vi "N6705b_Emulating_Mode_CCLOAD_Set_Current_limit.vi"(8 "error in (no error)":errorcluster {"code" format="%.0x"}, 9 "Dischage - Range":T1(ring), 10 "Limit (0.0 amps)":dbl=-0.013 format="%#_13g", 11 "VISA Refnum in":refnum<visa-resource-name>) -> (0 "error out":errorcluster {"code" format="%.0x"}, 3 "VISA Refnum out":refnum<visa-resource-name>)   [LabVIEW 2015]
uses:
  <instrlib>/Agilent N6700 Series/Agilent N6700 Series.lvlib
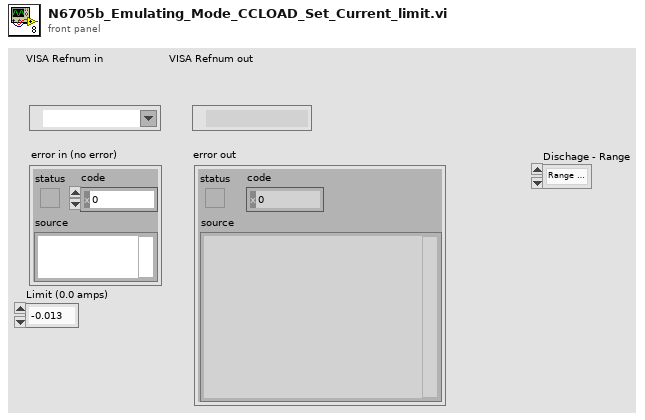
[diagram p1: front panel]
types:
  T1 = enum16{"Range 1 - 306mA", "Range 2 - 1.02 A", "Range 3 -  3.06"}
  T2 = enum16{"2 Quad Power Supply", "Unipower Supply", "CC Load", "CV Load", "VM", "CM"}
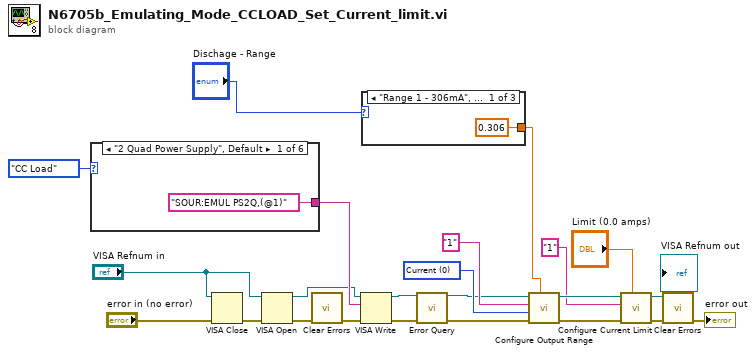
[diagram p0: block diagram]
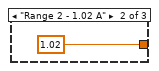
[diagram p2: hidden frame]
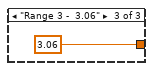
[diagram p3: hidden frame]
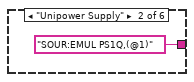
[diagram p4: hidden frame]
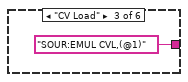
[diagram p5: hidden frame]
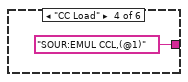
[diagram p6: hidden frame]
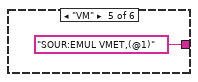
[diagram p7: hidden frame]
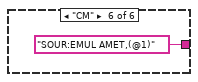
[diagram p8: hidden frame]
diagram:
  w17 = 0 items=["Voltage"=1, "Current"=0] ("Range Type (1: Voltage)")
  n1 = case shown="\"2 Quad Power Supply\", Default" T2."CC Load" ("Mode") {
    tunnel: ["SOUR:EMUL PS2Q,(@1)" ("write buffer") "SOUR:EMUL PS1Q,(@1)" ("write buffer") "SOUR:EMUL CVL,(@1)" ("write buffer") "SOUR:EMUL CCL,(@1)" ("write buffer") "SOUR:EMUL VMET,(@1)" ("write buffer") "SOUR:EMUL AMET,(@1)" ("write buffer")] -> w10
    frame "2 Quad Power Supply", Default {
    }
    frame "Unipower Supply" {
    }
    frame "CV Load" {
    }
    frame "CC Load" {
    }
    frame "VM" {
    }
    frame "CM" {
    }
  }
  n2 = VISA Close(VISA resource name="VISA Refnum in", error in (no error)="error in (no error)") -> (error out=w8:errorcluster)
  n3 = VISA Open(error in (no error)=w8, VISA resource name="VISA Refnum in") -> (VISA resource name=w3:refnum<visa-resource-name>, error out=w4:errorcluster)  [unwired: 3 in]
  n4 = call <vilib>:"Clear Errors.vi"("error in (no error)"=w4) -> ("error out"=w5:errorcluster)  [unwired: 5 in, 1 out]
  n5 = VISA Write(VISA resource name=w3, write buffer=w10, error in (no error)=w5) -> (VISA resource name out=w11:refnum<visa-resource-name>, error out=w12:errorcluster)  [unwired: 1 out]
  n6 = case shown="\"Range 1 - 306mA\", Default" "Dischage - Range" {
    tunnel: [0.306 ("Range (0.0)") 1.02 ("Range (0.0)") 3.06 ("Range (0.0)")] -> w1
    frame "Range 1 - 306mA", Default {
    }
    frame "Range 2 - 1.02 A" {
    }
    frame "Range 3 -  3.06" {
    }
  }
  n7 = call <instrlib>:"Error Query.vi"("VISA resource name"=w11, "error in (no error)"=w12) -> ("VISA resource name out"=w15:refnum<visa-resource-name>, "error out"=w21:errorcluster)  [unwired: 10 in, 2 out]
  n8 = call <instrlib>:"Configure Output Range.vi"("Range (0.0)"=w1, "error in (no error)"=w21, "Range Type (1: Voltage)"=w17, "Channel Name (1)"="1", "VISA resource name"=w15) -> ("error out"=w20:errorcluster, "VISA resource name out"=w18:refnum<visa-resource-name>)  [unwired: 5 in]
  n9 = call <instrlib>:"Configure Current Limit.vi"("Limit (0.0 amps)"="Limit (0.0 amps)", "error in (no error)"=w20, "Channel Name (1)"="1", "VISA resource name"=w18) -> ("error out"=w19:errorcluster, "VISA resource name out"=→"VISA Refnum out":refnum<visa-resource-name>)  [unwired: 6 in]
  n10 = call <vilib>:"Clear Errors.vi"("error in (no error)"=w19) -> ("error out"=→"error out":errorcluster)  [unwired: 5 in, 1 out]
